vi "host_wait_for_scan.vi"(8 "error in (no error)":errorcluster) -> (0 "error out":errorcluster)   [LabVIEW 2021]
doc: "This VI initialize variables for command. The counter for move will reset to 0."
uses:
  core/host_global_vars.vi
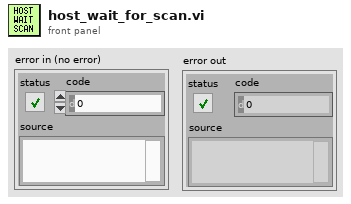
[diagram p1: front panel]
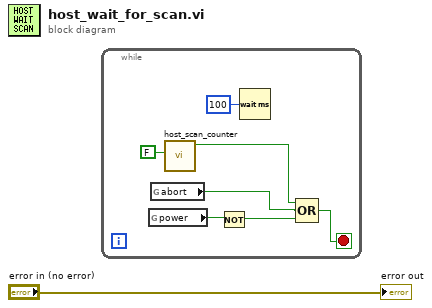
[diagram p0: block diagram]
diagram:
  n1 = while {
    stop <- w3 stop-if-true
    n2 = global read "host_global_vars.vi" "power"() -> (w7:bool)
    n3 = global read "host_global_vars.vi" "abort"() -> (w5:bool)
    n4 = call "host_scan_counter.vi"("update?"=FALSE) -> ("finished?"=w6:bool)  [unwired: 10 in]
    n5 = Not(x=w7) -> (.not. x?=w4:bool)
    n6 = Wait (ms)(milliseconds to wait=u32 100) -> ()  [unwired: 1 out]
    n7 = Compound Arithmetic op=OR(w6, w5, w4) -> (w3:bool)
  }
  "error out" <- "error in (no error)"
